vi "trataMsg.vi"(0 "addr":u8 format="%.0x", 7 "opcode":u8 format="%.0x", 11 "dado":u16 format="%.0x", 13 "ClusterUI":T1) -> ()   [LabVIEW 2018]
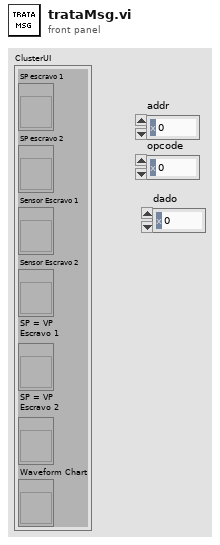
[diagram p1: front panel]
types:
  T1 = cluster{"SP escravo 1":refnum<vi>, "SP escravo 2":refnum<vi>, "Sensor Escravo 1":refnum<vi>, "Sensor Escravo 2":refnum<vi>, "SP = VP\nEscravo 1":refnum<vi>, "SP = VP\nEscravo 2":refnum<vi>, "Waveform Chart":refnum<vi>}
  T2 = cluster{"plot 0":dbl, "plot 1":dbl, "plot 2":dbl, "plot 3":dbl}
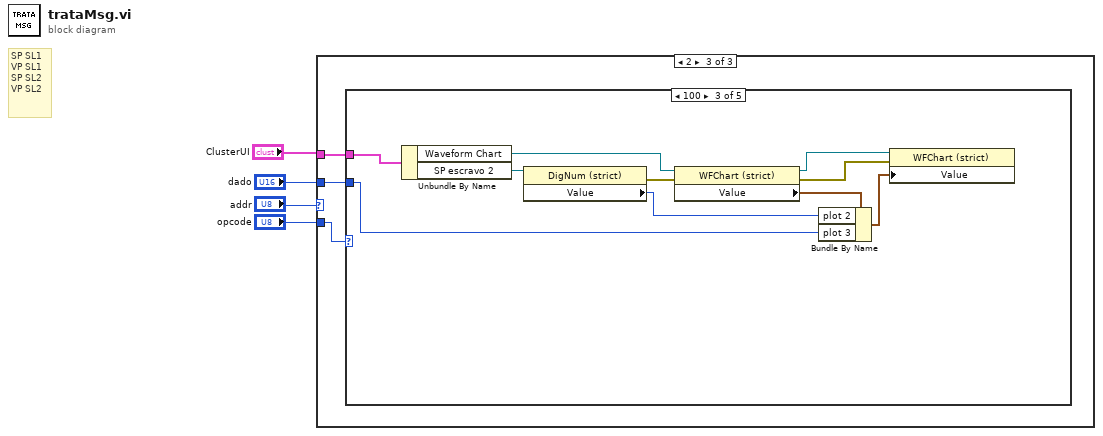
[diagram p0: block diagram]
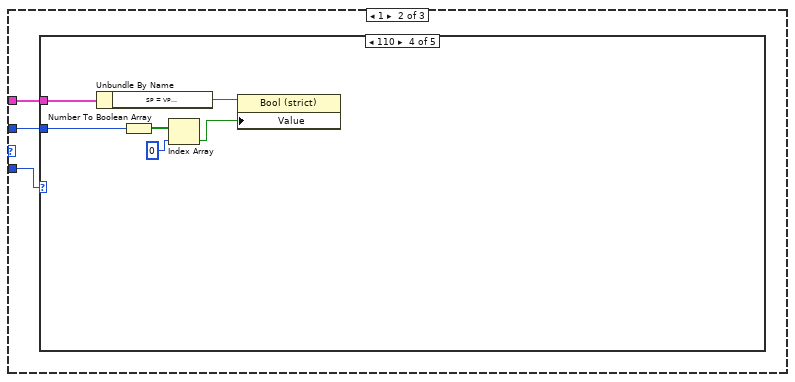
[diagram p3: hidden frame]
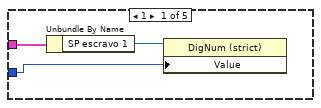
[diagram p4: hidden frame]
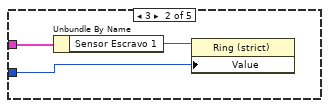
[diagram p5: hidden frame]
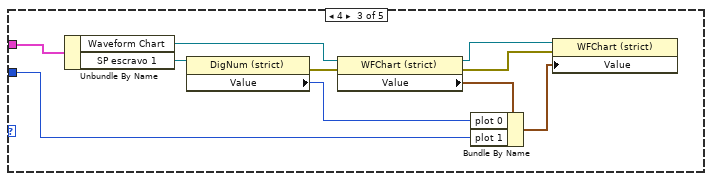
[diagram p6: hidden frame]
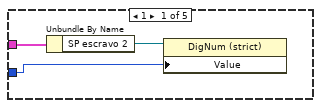
[diagram p8: hidden frame]
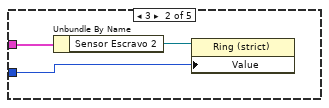
[diagram p9: hidden frame]
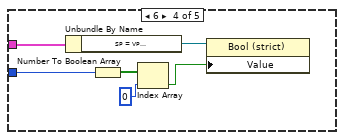
[diagram p10: hidden frame]
diagram:
  # "SP SL1\nVP SL1\nSP SL2\nVP SL2"
  n1 = case shown="2" "addr" {
    tunnel: "opcode" -> [_ w7 w30]
    tunnel: "dado" -> [_ w6 w31]
    tunnel: "ClusterUI" -> [_ w5 w32]
    frame 0, Default {
    }
    frame 1 {
      n2 = case shown="110" w7 {
        tunnel: w6 -> [w8 w11 w14 w27 _]
        tunnel: w5 -> [w10 w12 w23 w28 _]
        frame 1 {
          n3 = Unbundle By Name(w10) -> ("SP escravo 1"=w9:refnum<vi>)
          n4 = property class="DigNum (strict)"(reference=w9, "Value"=w8) -> ()  [unwired: 1 in, 2 out]
        }
        frame 3 {
          n5 = Unbundle By Name(w12) -> ("Sensor Escravo 1"=w13:refnum<vi>)
          n6 = property class="Ring (strict)"(reference=w13, "Value"=w11) -> ()  [unwired: 1 in, 2 out]
        }
        frame 4 {
          n7 = Unbundle By Name(w23) -> ("Waveform Chart"=w20:refnum<vi>, "SP escravo 1"=w22:refnum<vi>)
          n8 = property class="DigNum (strict)"(reference=w22) -> (error out=w21:errorcluster, "Value"=w15:u16)  [unwired: 1 in, 1 out]
          n9 = property class="WFChart (strict)"(reference=w20, error in=w21) -> (reference out=w19:refnum<vi>, error out=w18:errorcluster, "Value"=w17:T2)
          n10 = Bundle By Name(cluster=w17, "plot 0"=w15, "plot 1"=w14) -> (w16:T2)
          n11 = property class="WFChart (strict)"(reference=w19, error in=w18, "Value"=w16) -> ()  [unwired: 2 out]
        }
        frame 6 {
          n12 = Unbundle By Name(w28) -> ("SP = VP\nEscravo 1"=w29:refnum<vi>)
          n13 = Number To Boolean Array(number=w27) -> (Boolean array=w26:bool[])
          n14 = Index Array(array=w26, index=0) -> (element=w25:bool)
          n15 = property class="Bool (strict)"(reference=w29, "Value"=w25) -> ()  [unwired: 1 in, 2 out]
        }
        frame 7, Default {
        }
      }
    }
    frame 2 {
      n16 = case shown="100" w30 {
        tunnel: w31 -> [w33 w36 w40 w52 _]
        tunnel: w32 -> [w35 w37 w48 w53 _]
        frame 1 {
          n17 = Unbundle By Name(w35) -> ("SP escravo 2"=w34:refnum<vi>)
          n18 = property class="DigNum (strict)"(reference=w34, "Value"=w33) -> ()  [unwired: 1 in, 2 out]
        }
        frame 3 {
          n19 = Unbundle By Name(w37) -> ("Sensor Escravo 2"=w38:refnum<vi>)
          n20 = property class="Ring (strict)"(reference=w38, "Value"=w36) -> ()  [unwired: 1 in, 2 out]
        }
        frame 4 {
          n21 = Unbundle By Name(w48) -> ("Waveform Chart"=w45:refnum<vi>, "SP escravo 2"=w47:refnum<vi>)
          n22 = property class="DigNum (strict)"(reference=w47) -> (error out=w46:errorcluster, "Value"=w39:u16)  [unwired: 1 in, 1 out]
          n23 = property class="WFChart (strict)"(reference=w45, error in=w46) -> (reference out=w44:refnum<vi>, error out=w43:errorcluster, "Value"=w42:T2)
          n24 = Bundle By Name(cluster=w42, "plot 2"=w39, "plot 3"=w40) -> (w41:T2)
          n25 = property class="WFChart (strict)"(reference=w44, error in=w43, "Value"=w41) -> ()  [unwired: 2 out]
        }
        frame 6 {
          n26 = Unbundle By Name(w53) -> ("SP = VP\nEscravo 2"=w54:refnum<vi>)
          n27 = Number To Boolean Array(number=w52) -> (Boolean array=w51:bool[])
          n28 = Index Array(array=w51, index=0) -> (element=w50:bool)
          n29 = property class="Bool (strict)"(reference=w54, "Value"=w50) -> ()  [unwired: 1 in, 2 out]
        }
        frame 7, Default {
        }
      }
    }
  }
